vi "get_center.vi"(8 "error in (no error)":errorcluster, 11 "Box in":refnum<class "Box.lvclass">) -> (0 "error out":errorcluster, 2 "center":refnum<class "SpaceVector.lvclass">, 3 "Box out":refnum<class "Box.lvclass">)   [LabVIEW 2010, in "Box.lvclass"]
uses:
  Box.lvclass
  SpaceVector/SpaceVector/SpaceVector.lvclass
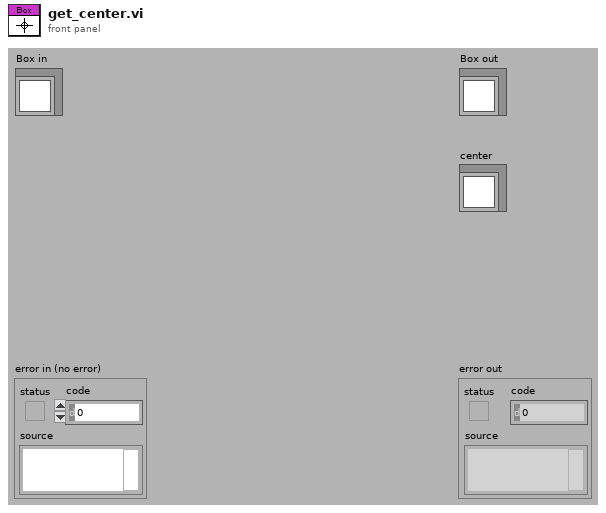
[diagram p1: front panel]
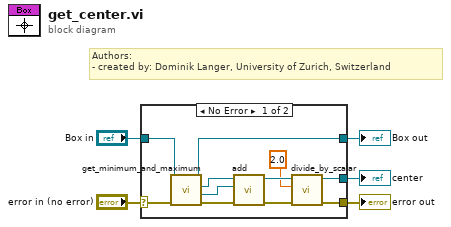
[diagram p0: block diagram]
diagram:
  # "Authors: \n- created by: Dominik Langer, University of Zurich, Switzerland"
  n1 = case shown="No Error" "error in (no error)" {
    selector: "error in (no error)" -> [w16 w18]
    tunnel: [w7 w18] -> w4
    tunnel: [w14 w17] -> w2
    tunnel: "Box in" -> [w15 w17]
    tunnel: [w6 _] -> w1
    frame No Error {
      n2 = call "get_minimum_and_maximum.vi"("error in (no error)"=w16, "Box in"=w15) -> ("error out"=w11:errorcluster, "maximum"=w12:refnum<class "SpaceVector.lvclass">, "minimum"=w13:refnum<class "SpaceVector.lvclass">, "Box out"=w14:refnum<class "Box.lvclass">)  [unwired: 6 in]
      n3 = call "add.vi"("error in (no error)"=w11, "vector to be added"=w12, "SpaceVector in"=w13) -> ("error out"=w8:errorcluster, "SpaceVector out"=w10:refnum<class "SpaceVector.lvclass">)  [unwired: 7 in]
      n4 = call "divide_by_scalar.vi"("error in (no error)"=w8, "divisor"=2.0, "SpaceVector in"=w10) -> ("error out"=w7:errorcluster, "SpaceVector out"=w6:refnum<class "SpaceVector.lvclass">)  [unwired: 7 in]
    }
    frame Error {
    }
  }
  "error out" <- w4
  "Box out" <- w2
  "center" <- w1
